vi "debuglog2.vi"(10 "Enum":enum16{"update", "init"}(ring), 11 "Log data":string) -> ()   [LabVIEW 2017]
uses:
  <vilib>/Utility/sysdir.llb/System Directory Type.ctl
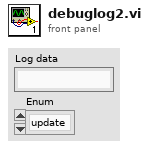
[diagram p1: front panel]
types:
  T1 = typedef "System Directory Type.ctl" = i32
  T2 = enum16{"open", "replace", "create", "open or create", "replace or create", "replace or create with confirmation"}
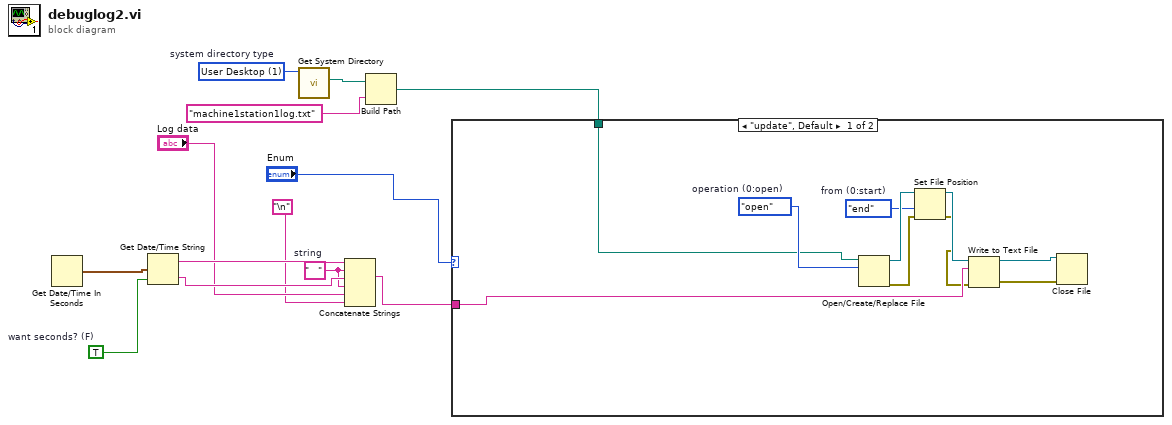
[diagram p0: block diagram]
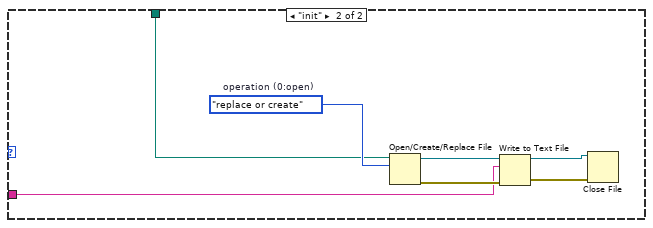
[diagram p2: hidden frame]
diagram:
  w1 = TRUE  # want seconds? (F)
  w6 = T1 1 items=["User Home"=0, "User Desktop"=1, "User Documents"=2, "User Application Data"=3, "User Preferences"=4, "User Temporary"=5, "Public Documents"=6, "Public Application Data"=7, "Public Preferences"=8, "Public Cache"=13, "System Core Libraries"=9, "System Installed Libraries"=10, "Application Files"=11, "Boot Volume Root"=12]  # system directory type
  w10 = "   "  # string
  n1 = Get Date/Time In Seconds() -> (seconds since 1Jan1904=w13:timestamp)
  n2 = Get Date/Time String(seconds (now)=w13, want seconds? (F)=w1) -> (date string=w12:string, time string=w11:string)  [unwired: 1 in]
  n3 = call <vilib>:"Get System Directory.vi"("system directory type"=w6) -> ("system directory"=w8:path)  [unwired: 10 in]
  n4 = Concatenate Strings(w12, w10, w11, w10, "Log data", "\n") -> (w4:string)
  n5 = Build Path(base path=w8, name or relative path="machine1station1log.txt") -> (appended path=w5:path)
  n6 = case shown="\"update\", Default" "Enum" {
    tunnel: w5 -> [w20 w25]
    tunnel: w4 -> [w19 w24]
    frame "update", Default {
      w14 = enum16{"start", "end", "current"}."end"  # from (0:start)
      w21 = T2."open"  # operation (0:open)
      n7 = Open/Create/Replace File(file path (use dialog)=w20, operation (0:open)=w21) -> (refnum out=w18:refnum<file>, error out=w16:errorcluster)  [unwired: 4 in, 1 out]
      n8 = Set File Position(refnum=w18, from (0:start)=w14, error in=w16) -> (refnum out=w17:refnum<file>, error out=w15:errorcluster)  [unwired: 1 in]
      n9 = Write to Text File(file (use dialog)=w17, text=w19, error in=w15) -> (refnum out=w23:refnum<file>, error out=w22:errorcluster)  [unwired: 1 in, 1 out]
      n10 = Close File(refnum=w23, error in=w22) -> ()  [unwired: 2 out]
    }
    frame "init" {
      w30 = T2."replace or create"  # operation (0:open)
      n11 = Open/Create/Replace File(file path (use dialog)=w25, operation (0:open)=w30) -> (refnum out=w29:refnum<file>, error out=w26:errorcluster)  [unwired: 4 in, 1 out]
      n12 = Write to Text File(file (use dialog)=w29, text=w24, error in=w26) -> (refnum out=w28:refnum<file>, error out=w27:errorcluster)  [unwired: 1 in, 1 out]
      n13 = Close File(refnum=w28, error in=w27) -> ()  [unwired: 2 out]
    }
  }
